vi "ScopeScratch.vi"() -> ()   [LabVIEW 2021]
uses:
  Sources/Config_Cluster.ctl
  Sources/Mode_Enum.ctl
panel:
  out "Success?":bool
  out "message":string
  out "Response Value 2":dbl caption="Response Value" format="%.6f"
  out "Response Value":dbl format="%.6f"
  out "Measurement Result":dbl format="%^.3e"
  out "Acquisition Time":dbl format="%^.3e"
  out "Sample Rate":dbl format="%^.3e"
  out "Divisions":i32
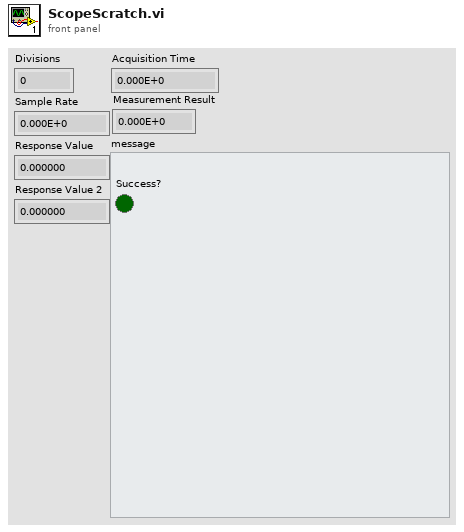
[diagram p1: front panel]
types:
  T1 = typedef "Config_Cluster.ctl" = cluster{"General":cluster{"Config.ini":path, "Default Logging Path":path}, "Hardware":cluster{"Global T VAR":refnum<k21>, "Global B VAR":refnum<k21>, "VISAS":cluster{"GEN COM":refnum<visa-resource-name>, "SCOPE COM":refnum<visa-resource-name>, "VNA COM":refnum<visa-resource-name>}}, "Operation":cluster{"Operation Mode":T2, "Status":string, "NewLog?":bool, "OvenWarn":bool, "Scope Settings":cluster{"TimeBase":dbl, "VerticalScale":dbl}}}
  T2 = typedef "Mode_Enum.ctl" = enum16{"OvenNRDY", "Logging", "Idle-Off", "Idle"}
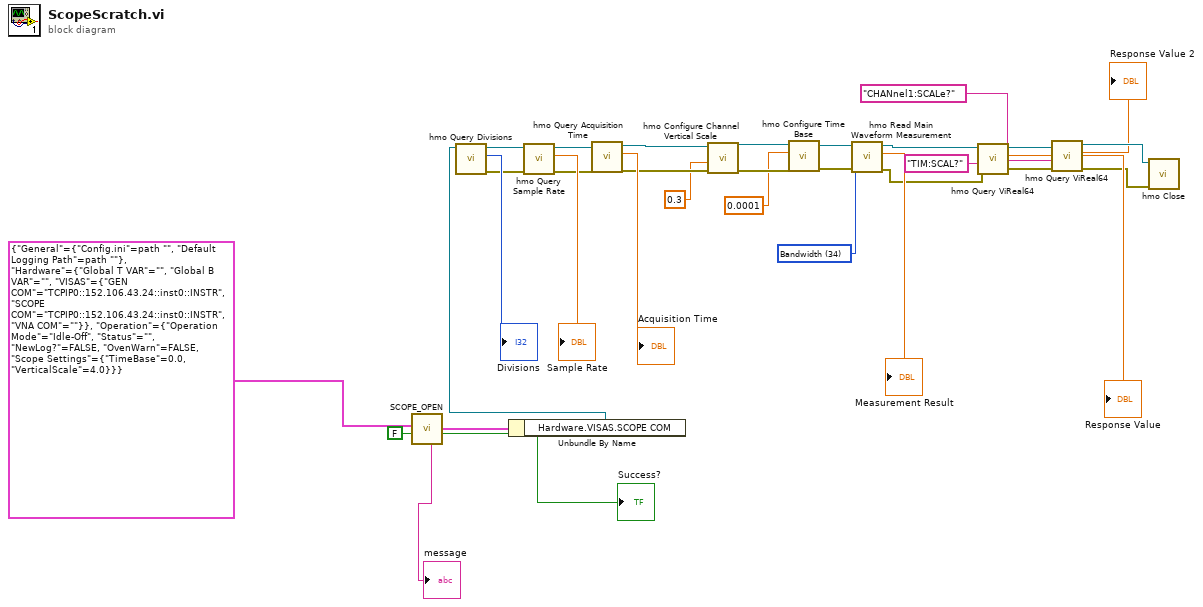
[diagram p0: block diagram]
diagram:
  w18 = 34 items=["Frequency"=1, "Period"=2, "Peak Peak"=3, "Peak Upper"=4, "Peak Lower"=5, "Positive Pulses Count"=6, "Negative Pulses Count"=7, "Rising Edges Count"=8, "Falling Edges Count"=9, "High"=10, "Low"=11, "Amplitude"=12, "Mean Value"=13, "RMS Value"=14, "Rise Time"=15, "Falling Time"=16, "Duty Cycle Positive"=17, "Duty Cycle Negative"=18, "Pulse Width Positive"=19, "Pulse Width Negative"=20, "Cycle Mean"=21, "Cycle RMS"=22, "Standard Deviation"=23, "Trigger Frequency"=24, "Trigger Period"=25, "Positive Overshoot"=26, "Negative Overshoot"=27, "Delay"=28, "Phase"=29, "Waveform Mean"=30, "Waveform RMS"=31, "Waveform Standard Deviation"=32, "Cycle Standard Deviation"=33, "Bandwidth"=34, "Crest Factor"=35] ("Measurement Function (Frequency)")
  n1 = call "SCOPE_OPEN.vi"("Clear Error w/ Report?"=FALSE, "Configuration Cluster"=T1 {"General"={"Config.ini"=path "", "Default Logging Path"=path ""}, "Hardware"={"Global T VAR"="", "Global B VAR"="", "VISAS"={"GEN COM"="TCPIP0::152.106.43.24::inst0::INSTR", "SCOPE COM"="TCPIP0::152.106.43.24::inst0::INSTR", "VNA COM"=""}}, "Operation"={"Operation Mode"=enum."Idle-Off", "Status"="", "NewLog?"=FALSE, "OvenWarn"=FALSE, "Scope Settings"={"TimeBase"=0.0, "VerticalScale"=4.0}}}) -> ("Success?"=→"Success?":bool, "Configuration Cluster Out"=w3:T1, "message"=→"message":string)  [unwired: 6 in, 1 out]
  n2 = Unbundle By Name(w3) -> ("Hardware.VISAS.SCOPE COM"=w2:refnum<visa-resource-name>)
  n3 = call <instrlib>:"hmo Query Divisions.vi"("VISA resource name"=w2) -> ("error out"=w31:errorcluster, "Divisions"=→"Divisions":i32, "VISA resource name out"=w32:refnum<visa-resource-name>)  [unwired: 8 in]
  n4 = call <instrlib>:"hmo Query Sample Rate.vi"("error in (no error)"=w31, "VISA resource name"=w32) -> ("error out"=w28:errorcluster, "Sample Rate"=→"Sample Rate":dbl, "VISA resource name out"=w29:refnum<visa-resource-name>)  [unwired: 7 in]
  n5 = call <instrlib>:"hmo Query Acquisition Time.vi"("error in (no error)"=w28, "VISA resource name"=w29) -> ("error out"=w25:errorcluster, "Acquisition Time"=→"Acquisition Time":dbl, "VISA resource name out"=w26:refnum<visa-resource-name>)  [unwired: 7 in]
  n6 = call <instrlib>:"hmo Configure Channel Vertical Scale.vi"("error in (no error)"=w25, "Vertical Scale (0.005)"=0.3, "VISA resource name"=w26) -> ("error out"=w22:errorcluster, "VISA resource name out"=w23:refnum<visa-resource-name>)  [unwired: 7 in]
  n7 = call <instrlib>:"hmo Configure Time Base.vi"("error in (no error)"=w22, "Time Scale (100.0e-6)"=0.0001, "VISA resource name"=w23) -> ("error out"=w20:errorcluster, "VISA resource name out"=w19:refnum<visa-resource-name>)  [unwired: 7 in]
  n8 = call <instrlib>:"hmo Read Main Waveform Measurement.vi"("error in (no error)"=w20, "Measurement Function (Frequency)"=w18, "VISA resource name"=w19) -> ("error out"=w14:errorcluster, "Measurement Result"=→"Measurement Result":dbl, "VISA resource name out"=w15:refnum<visa-resource-name>)  [unwired: 6 in]
  n9 = call <instrlib>:"hmo Query ViReal64.vi"("error in (no error)"=w14, "Query"="TIM:SCAL?", "VISA resource name"=w15) -> ("error out"=w11:errorcluster, "Response Value"=→"Response Value":dbl, "VISA resource name out"=w12:refnum<visa-resource-name>)  [unwired: 6 in]
  n10 = call <instrlib>:"hmo Query ViReal64.vi"("error in (no error)"=w11, "Query"="CHANnel1:SCALe?", "VISA resource name"=w12) -> ("error out"=w10:errorcluster, "Response Value"=→"Response Value 2":dbl, "VISA resource name out"=w9:refnum<visa-resource-name>)  [unwired: 6 in]
  n11 = call <instrlib>:"hmo Close.vi"("error in (no error)"=w10, "VISA resource name"=w9) -> ()  [unwired: 9 in, 1 out]
